vi "CreateClass.vi"(7 "PythonConverter_BD in":refnum<class "PyConvBD.lvclass">, 8 "error in":errorcluster, 11 "ForLoop in":refnum<class "ForLoop.lvclass">) -> (0 "error out":errorcluster, 3 "ForLoop out":refnum<class "ForLoop.lvclass">, 4 "class":string, 5 "PythonConverter_BD out":refnum<class "PyConvBD.lvclass">)   [LabVIEW 2014, in "ForLoop.lvclass"]
uses:
  ForLoop.lvclass
  Python/PythonConverter_BD/PyConvBD.lvclass
  Structure/Structure.lvclass/Structure.ctl
  Diagram/Diagram.lvclass
  Python/Parsing/Python Functions.lvlib
  Structure/Structure.lvclass
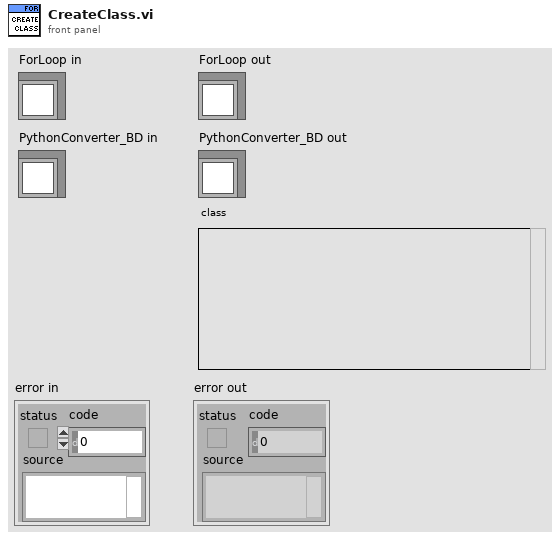
[diagram p1: front panel]
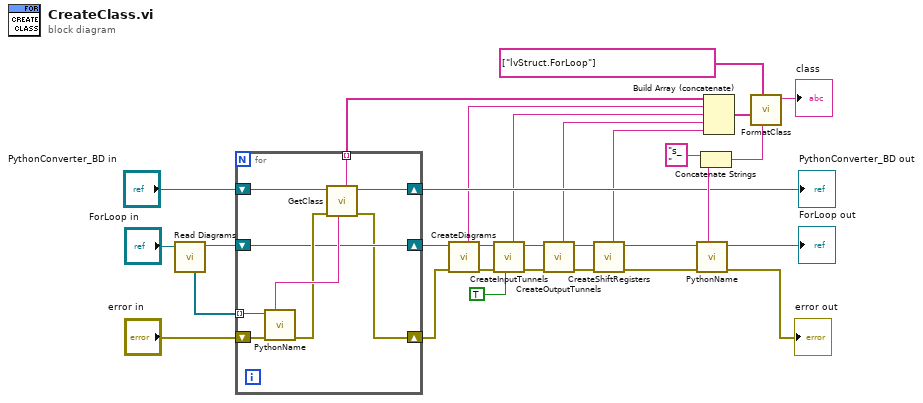
[diagram p0: block diagram]
diagram:
  n1 = call "Read Diagrams.vi"("Structure in"="ForLoop in") -> ("Structure out"=w23:refnum<class "ForLoop.lvclass">, "Diagrams"=w25:refnum<class "Diagram.lvclass">[])  [unwired: 7 in]
  n2 = for {
    tunnel: w25 -> [w39] mode=indexing
    shift-right: [w34] -> w22
    shift-left: "PythonConverter_BD in" -> [w38]
    shift-right: [w35] -> w21
    shift-left: w23 -> [w35]
    tunnel: [w33] -> w16 mode=indexing
    shift-right: [w31] -> w17
    shift-left: "error in" -> [w32]
    n3 = call-dynamic "PythonName.vi"("error in"=w32, "Diagram in"=w39) -> ("error out"=w36:errorcluster, "UID"=w37:string)  [unwired: 6 in, 2 out]
    n4 = call "GetClass.vi"("name"=w37, "error in"=w36, "PythonConverter_BD in"=w38) -> ("error out"=w31:errorcluster, "PythonConverter_BD out"=w34:refnum<class "PyConvBD.lvclass">, "class"=w33:string)  [unwired: 4 in]
  }
  "PythonConverter_BD out" <- w22
  n5 = call-dynamic "CreateDiagrams.vi"("error in"=w17, "ForLoop in"=w21) -> ("error out"=w11:errorcluster, "ForLoop out"=w12:refnum<class "ForLoop.lvclass">, "create_diagrams"=w15:string)  [unwired: 5 in]
  n6 = call-dynamic "CreateInputTunnels.vi"("controlling"=TRUE, "error in"=w11, "Loop in"=w12) -> ("error out"=w8:errorcluster, "Loop out"=w9:refnum<class "ForLoop.lvclass">, "createTunnels"=w10:string)  [unwired: 4 in]
  n7 = call-dynamic "CreateOutputTunnels.vi"("error in"=w8, "Loop in"=w9) -> ("error out"=w5:errorcluster, "Loop out"=w6:refnum<class "ForLoop.lvclass">, "createTunnels"=w7:string)  [unwired: 5 in]
  n8 = call-dynamic "CreateShiftRegisters.vi"("error in"=w5, "Loop in"=w6) -> ("error out"=w3:errorcluster, "Loop out"=w4:refnum<class "ForLoop.lvclass">, "createSR"=w2:string)  [unwired: 5 in]
  n9 = call-dynamic "PythonName.vi"("error in"=w3, "Node in"=w4) -> ("error out"=→"error out":errorcluster, "Node out"=→"ForLoop out":refnum<class "ForLoop.lvclass">, "UID"=w28:string)  [unwired: 6 in, 1 out]
  n10 = Concatenate Strings("s_" ("format string"), w28) -> (w27:string)
  n11 = Build Array (concatenate)(w16, w15, w10, w7, w2) -> (w14:string[])
  n12 = call "FormatClass.vi"("name"=w27, "parameters/ancestors"=string[] ["lvStruct.ForLoop"], "body"=w14) -> ("python"=→"class":string)  [unwired: 8 in]
